vi "Q -- interval count.vi"(6 "interval (sec)":dbl=nan, 8 "last time (sec)":dbl=nan, 10 "current time (sec)":dbl) -> (0 "last time out (sec)":dbl=nan, 1 "time since last tic (sec)":dbl=nan, 2 "tic state":enum16{"knock-knock", "none"}(ring), 3 "tic":bool)   [LabVIEW 2015]
uses:
  Q - not nan -- real.vi
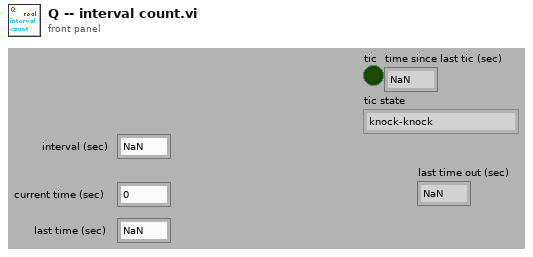
[diagram p1: front panel]
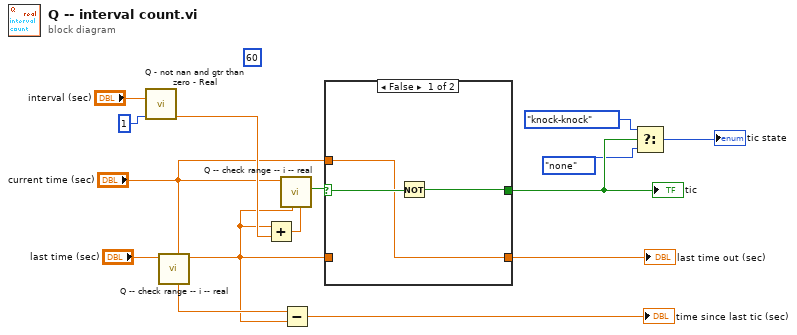
[diagram p0: block diagram]
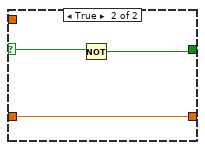
[diagram p2: hidden frame]
diagram:
  (unwired) 60 ("y")
  n1 = call "Q - not nan and gtr than zero - Real.vi"("default"=1 ("y"), "Numeric"="interval (sec)") -> ("out"=w12:dbl)  [unwired: 8 in, 1 out]
  n2 = call "Q -- check range -- i -- real.vi"("upper"="current time (sec)", "number"="last time (sec)") -> ("number in range"=w6:dbl)  [unwired: 7 in, 2 out]
  n3 = Add(x=w6, y=w12) -> (x+y=w11:dbl)
  n4 = call "Q -- check range -- i -- real.vi"("upper"=w11, "lower"=w6, "number"="current time (sec)") -> ("in range?"=w10:bool)  [unwired: 6 in, 2 out]
  n5 = Subtract(x="current time (sec)", y=w6) -> (x-y=→"time since last tic (sec)":dbl)
  n6 = case shown="False" w10 {
    selector: w10 -> [w17 w20]
    tunnel: [w16 w19] -> w4
    tunnel: [w15 w18] -> w9
    tunnel: "current time (sec)" -> [w15 _]
    tunnel: w6 -> [_ w18]
    frame False {
      n7 = Not(x=w17) -> (.not. x?=w16:bool)
    }
    frame True {
      n8 = Not(x=w20) -> (.not. x?=w19:bool)
    }
  }
  "tic" <- w4
  "last time out (sec)" <- w9
  n9 = Select(t=enum16{"knock-knock", "none"}."knock-knock" ("state"), s=w4, f=enum16{"knock-knock", "none"}."none" ("state")) -> (s? t:f=→"tic state":enum16{"knock-knock", "none"})
